vi "Read Lossy.vi"(3 "Wait for Next? (F)":bool, 4 "Connection":refnum<class "Connection.lvclass">, 5 "Wait Timeout mS (-1)":i32=-1) -> (0 "Closed?":bool, 1 "Element":T1, 2 "Timed Out?":bool)   [LabVIEW 2020, in "Connection.lvclass"]
uses:
  Connection.lvclass
  Element.ctl
  Connection.lvclass/Connection.ctl
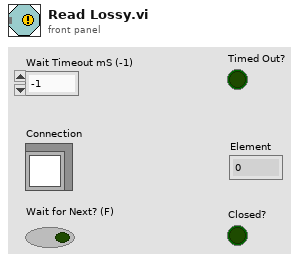
[diagram p1: front panel]
types:
  T1 = typedef "Connection.lvclass/Element.ctl" = dbl
  T2 = typedef "Connection.lvclass/Tag Data.ctl" = cluster{"Value":T1, "Updated":timestamp, "Sequence":u32}
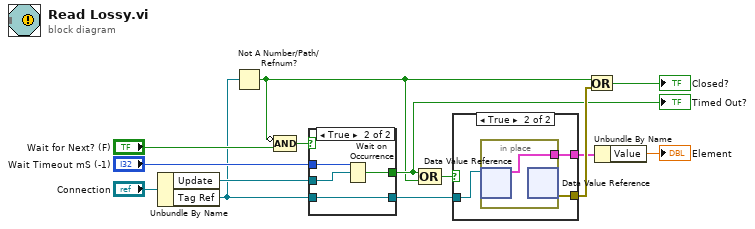
[diagram p0: block diagram]
diagram:
  n1 = Unbundle By Name("Connection") -> ("Update"=w10:refnum<k4>, "Tag Ref"=w8:refnum<data-value>)
  n2 = Not A Number/Path/Refnum?(number/path/refnum=w8) -> (NaN/Path/Refnum?=w3:bool)
  n3 = Compound Arithmetic op=AND(invert w3, "Wait for Next? (F)") -> (w11:bool)
  n4 = case shown="True" w11 {
    tunnel: w10 -> [_ w19]
    tunnel: "Wait Timeout mS (-1)" -> [_ w18]
    tunnel: w8 -> [w15 w17]
    tunnel: [w15 w17] -> w7
    tunnel: [_ w16] -> w5
    frame False {
    }
    frame True {
      n5 = Wait on Occurrence(2:w19, 3:w18) -> (0:w16:bool)  [unwired: 1 in]
    }
  }
  "Timed Out?" <- w5
  n6 = Compound Arithmetic op=OR(w5, w3) -> (w6:bool)
  n7 = case shown="True" w6 {
    tunnel: w7 -> [_ w22]
    tunnel: [_ w21] -> w2
    tunnel: [_ w20] -> w14
    frame False {
    }
    frame True {
      n8 = in-place {
        in-place-border: [w23] -> w21
        n9 = in-place-dvr #1(w22) -> (w23:T2)  [unwired: 1 out]
        n10 = in-place-dvr #1() -> (w20:errorcluster)  [unwired: 1 in, 1 out]
      }
    }
  }
  n11 = Or(x=w3, y=w14) -> (x .or. y?=→"Closed?":bool)
  n12 = Unbundle By Name(w2) -> ("Value"=→"Element":T1)
